vi "Periodic Tasks.vi"(8 "error in":errorcluster) -> ()   [LabVIEW 2014]
doc: "This VI runs in parallel to other tasks. It can contain as many user-defined periodic loops as you need. These can carry out PID or other sorts of timed response."
uses:
  <vilib>/Rock Robotics/WPI/Joystick/WPI_JoystickGetSetRefNum.vi
  Robot Global Data.vi
  <vilib>/Rock Robotics/Network Tables/SD Write Boolean.vi
  <vilib>/Rock Robotics/Network Tables/SD Write Number.vi
  SimpleGyro/SimpleGyro.lvlib
panel:
  out "ARI Output Controls":T1
  out "Lifter Status":T2
  in  "Front Lift Joystick Values":T3
  in  "ARI Input Controls":T1
  out "LaunchPad Buttons":bool[](array[boolean])
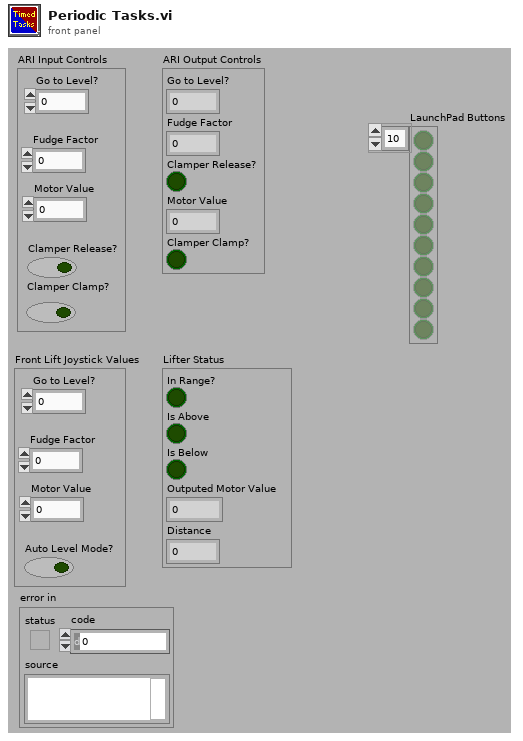
[diagram p1: front panel]
types:
  T1 = cluster{"Go to Level?":i32, "Fudge Factor":dbl, "Clamper Release?":bool, "Motor Value":dbl, "Clamper Clamp?":bool}
  T2 = cluster{"In Range?":bool, "Is Above":bool, "Is Below":bool, "Outputed Motor Value":dbl, "Distance":dbl}
  T3 = cluster{"Go to Level?":i32, "Fudge Factor":dbl, "Auto Level Mode?":bool, "Motor Value":dbl}
  T4 = typedef "WPI_JoystickDevRef.ctl" = cluster{"Device":T5}
  T5 = typedef "WPI_JoystickDeviceEnum.ctl" = enum16{"USB 0", "USB 1", "USB 2", "USB 3", "USB 4", "USB 5"}
  T6 = typedef "WPI_MotorControlDeviceRef.ctl" = cluster{"DeviceStatus":errorcluster, "Type":T7, "PWM":cluster{"Controller":T8, "PWM Channel":T9, "DeadBand":T10}, "CAN":cluster{"Device Number":u8, "Control Mode":T11, "Semaphore":T12, "Max Vout":dbl, "TalonSRX Control Mode":T13}, "Invert":bool, "TransformRef":T14, "InvTransformRef":T14}
  T7 = typedef "WPI_MotorControlType.ctl" = enum16{"PWM", "CAN", "CANTalonSRX"}
  T8 = typedef "FPGA_TypedefDigitalModule.ctl" = enum16{"Controller 1"}
  T9 = typedef "FPGA_DIOPWMChannel.ctl" = enum8{"PWM 0", "PWM 1", "PWM 2", "PWM 3", "PWM 4", "PWM 5", "PWM 6", "PWM 7", "PWM 8", "PWM 9", "PWM MXP 0", "PWM MXP 1", "PWM MXP 2", "PWM MXP 3", "PWM MXP 4", "PWM MXP 5", "PWM MXP 6", "PWM MXP 7", "PWM MXP 8", "PWM MXP 9", "Invalid"}
  T10 = typedef "WPI_PWMDeadband.ctl" = cluster{"Name":string, "maxPositivePwm":i32, "minPositivePwm":i32, "centerPwm":i32, "maxNegativePwm":i32, "minNegativePwm":i32, "angularRange":u16}
  T11 = typedef "WPI_CANJaguar_ControlMode.ctl" = enum8{"Percent VBus", "Current", "Speed", "Position", "Voltage"}
  T12 = typedef "Semaphore RefNum" = refnum<k1>
  T13 = typedef "WPI_CANTalonSRX_APIControlMode.ctl" = enum8{"Percent VBus", "Speed", "Position", "Slave", "Unchanged / Invalid"}
  T14 = typedef "WPI_PWMTransform_ConPane.ctl" = refnum<vi>
  T15 = typedef "SimpleGyro.lvlib/WPI_SimpleGyroDevRef.ctl" = cluster{"DevStatus":errorcluster, "Handle":i32, "Controller":T8, "SPI Bus":T16, "Device Found":bool, "Sample Rate":dbl}
  T16 = typedef "spi_bus.ctl" = enum16{"SPI On-Board, CS0", "SPI On-Board, CS1", "SPI On-Board, CS2", "SPI On-Board, CS3", "SPI MXP", "Invalid"}
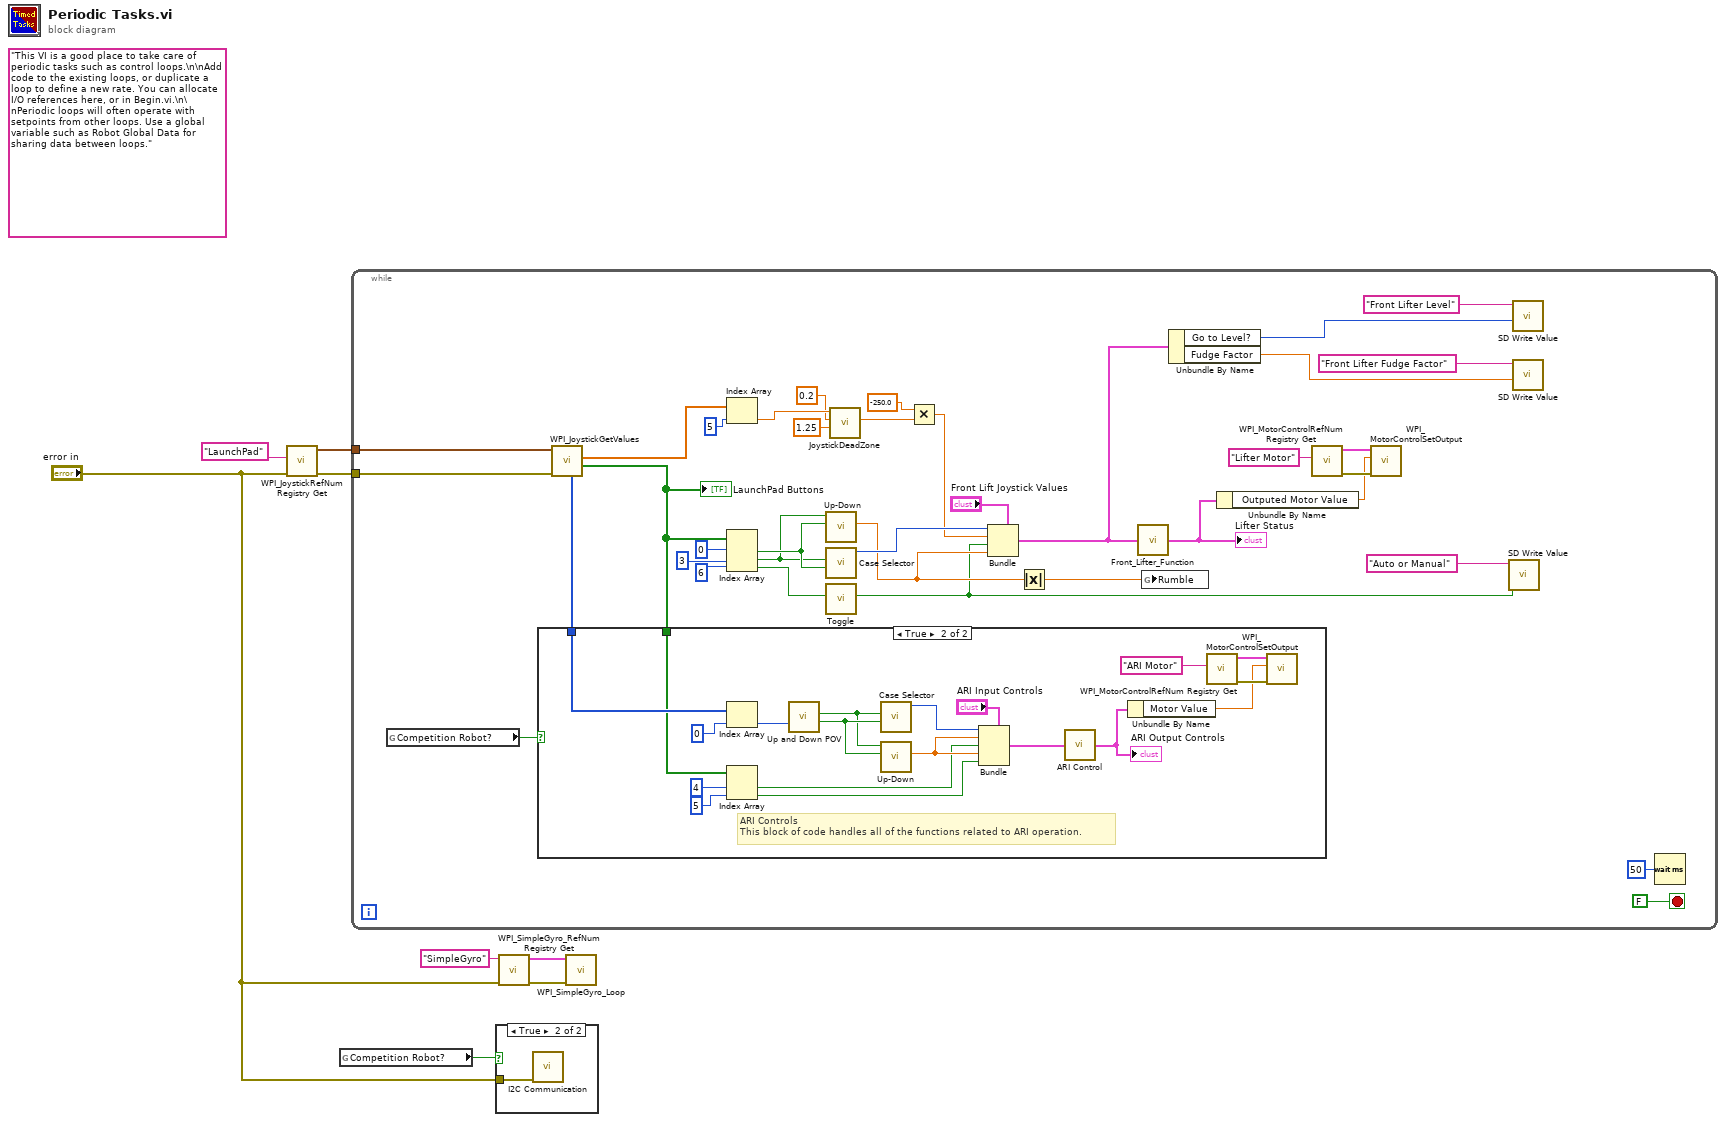
[diagram p0: block diagram]
diagram:
  (unwired) "This VI is a good place to take care of periodic tasks such as control loops.\n\nAdd code to the existing loops, or duplicate a loop to define a new rate. You can allocate I/O references here, or in Begin.vi.\n\nPeriodic loops will often operate with setpoints from other loops. Use a global variable such as Robot Global Data for sharing data between loops."
  n1 = call <vilib>:"WPI_JoystickRefNum Registry Get.vi"("error in (no error)"="error in", "refnum name"="LaunchPad") -> ("error out"=w6:errorcluster, "JoystickDevRef"=w7:T4)  [unwired: 8 in]
  n2 = global read "Robot Global Data.vi" "Competition Robot?"() -> (w1:bool)
  n3 = while {
    tunnel: w7 -> [w17]
    tunnel: w6 -> [w16]
    stop <- FALSE stop-if-true
    n4 = global read "Robot Global Data.vi" "Competition Robot?"() -> (w15:bool)
    n5 = call <vilib>:"WPI_JoystickGetValues.vi"("error in (no error)"=w16, "JoystickDevRef"=w17) -> ("Buttons"=w23:bool[], "Axes"=w29:dbl[], "POVs"=w39:i16[])  [unwired: 5 in, 2 out]
    "LaunchPad Buttons" <- w23
    n6 = case shown="True" w15 {
      tunnel: w39 -> [_ w59]
      tunnel: w23 -> [_ w51]
      frame False {
      }
      frame True {
        # "ARI Controls\nThis block of code handles all of the functions related to ARI operation."
        n7 = Index Array(array=w59, index=0) -> (element=w57:i16)
        n8 = Index Array(array=w51, index #1=4 ("index"), index #2=5 ("index")) -> (element #1=w53:bool, element #2=w52:bool)
        n9 = call "Up and Down POV.vi"("POV"=w57) -> ("Go Down?"=w62:bool, "Go Up?"=w56:bool)  [unwired: 9 in]
        n10 = call "Case Selector.vi"("Click Down"=w62, "Click Up"=w56) -> ("State"=w61:i32)  [unwired: 7 in, 2 out]
        n11 = call "Up-Down.vi"("Down"=w62, "Up"=w56) -> ("Direction"=w60:dbl)  [unwired: 9 in]
        n12 = Bundle(cluster="ARI Input Controls", "Go to Level?"=w61, "Fudge Factor"=w60, "Clamper Release?"=w53, "Motor Value"=w60, "Clamper Clamp?"=w52) -> (w63:T1)
        n13 = call "ARI Control.vi"("ARI Input Controls"=w63) -> ("ARI Output Controls"=w47:T1)  [unwired: 4 in]
        "ARI Output Controls" <- w47
        n14 = Unbundle By Name(w47) -> ("Motor Value"=w46:dbl)
        n15 = call <vilib>:"WPI_MotorControlRefNum Registry Get.vi"("refnum name"="ARI Motor") -> ("error out"=w49:errorcluster, "MotorControlDevRef"=w50:T6)  [unwired: 9 in]
        n16 = call <vilib>:"WPI_MotorControlSetOutput.vi"("error in (no error)"=w49, "Output"=w46, "MotorControlDevRef"=w50) -> ()  [unwired: 6 in, 3 out]
      }
    }
    n17 = Index Array(array=w29, index=5) -> (element=w22:dbl)
    n18 = Index Array(array=w23, index #1=0 ("index"), index #2=3 ("index"), index #3=6 ("index")) -> (element #1=w30:bool, element #2=w26:bool, element #3=w25:bool)
    n19 = call "Up-Down.vi"("Down"=w30, "Up"=w26) -> ("Direction"=w36:dbl)  [unwired: 9 in]
    n20 = call "Case Selector.vi"("Click Down"=w30, "Click Up"=w26) -> ("State"=w41:i32)  [unwired: 7 in, 2 out]
    n21 = call "Toggle.vi"("Input"=w25) -> ("Output"=w34:bool)  [unwired: 10 in]
    n22 = call "JoystickDeadZone.vi"("scale"=1.25, "dead zone"=0.2, "input variable"=w22) -> ("output variable"=w21:dbl)  [unwired: 8 in]
    n23 = Multiply(x=-250.0, y=w21) -> (x*y=w37:dbl)
    n24 = Bundle(cluster="Front Lift Joystick Values", "Go to Level?"=w41, "Fudge Factor"=w37, "Auto Level Mode?"=w34, "Motor Value"=w36) -> (w32:T3)
    n25 = Absolute Value(x=w36) -> (abs(x)=w14:dbl)
    n26 = call "Front_Lifter_Function.vi"("Joystick Values"=w32) -> ("Lifter Status"=w10:T2)  [unwired: 4 in]
    "Lifter Status" <- w10
    n27 = global write "Robot Global Data.vi" "Rumble"(w14) -> ()
    n28 = Unbundle By Name(w32) -> ("Go to Level?"=w18:i32, "Fudge Factor"=w40:dbl)
    n29 = Unbundle By Name(w10) -> ("Outputed Motor Value"=w9:dbl)
    n30 = call <vilib>:"WPI_MotorControlRefNum Registry Get.vi"("refnum name"="Lifter Motor") -> ("error out"=w11:errorcluster, "MotorControlDevRef"=w12:T6)  [unwired: 9 in]
    n31 = call <vilib>:"WPI_MotorControlSetOutput.vi"("error in (no error)"=w11, "Output"=w9, "MotorControlDevRef"=w12) -> ()  [unwired: 6 in, 3 out]
    n32 = call-poly <vilib>:"SD Write Value.vi"("Boolean"=w34, "Name"="Auto or Manual") -> ()  [unwired: 8 in, 2 out]
    n33 = call-poly <vilib>:"SD Write Value.vi"("Numeric"=w18, "Name"="Front Lifter Level") -> ()  [unwired: 8 in, 2 out]
    n34 = call-poly <vilib>:"SD Write Value.vi"("Numeric"=w40, "Name"="Front Lifter Fudge Factor") -> ()  [unwired: 8 in, 2 out]
    n35 = Wait (ms)(milliseconds to wait=u32 50) -> ()  [unwired: 1 out]
  }
  n36 = case shown="True" w1 {
    tunnel: "error in" -> [_ w65]
    frame False {
    }
    frame True {
      n37 = call "I2C Communication.vi"("error in"=w65) -> ()  [unwired: 11 in]
    }
  }
  n38 = call "WPI_SimpleGyro_RefNum Registry Get.vi"("error in (no error)"="error in", "refnum name"="SimpleGyro") -> ("error out"=w4:errorcluster, "SimpleGyroDevRef"=w5:T15)  [unwired: 8 in]
  n39 = call "WPI_SimpleGyro_Loop.vi"("error in"=w4, "SimpleGyroDevRef"=w5) -> ()  [unwired: 9 in, 1 out]
